vi "Write to Syslog.vi"(8 "error in (no error)":errorcluster, 10 "message":string, 11 "CIF Message Type":T1) -> (0 "error out":errorcluster)   [LabVIEW 2021, in "CIFLogs.lvlib"]
uses:
  CIFLogs.lvlib
  Typedef/Message Type.ctl
  <vilib>/CIF Foundation/CIF Utilities/Time/System Time/LabVIEW Time to TAI Time.vi
  Typedef/syslog facility.ctl
  Typedef/syslog priority.ctl
  <vilib>/CIF Foundation/CIF Utilities/Time/Time_CIF_U.lvlib
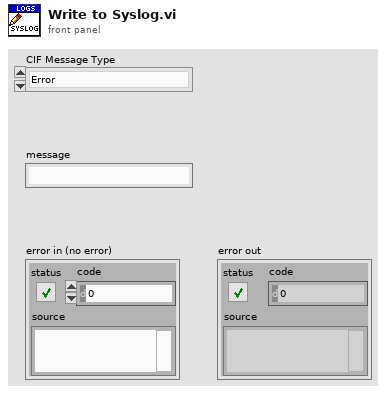
[diagram p1: front panel]
types:
  T1 = typedef "CIFLogs.lvlib/Message Type.ctl" = enum16{"Error", "Information", "Print Terminal", "Configuration"}
  T2 = typedef "CIFLogs.lvlib/syslog priority.ctl" = enum8{"emerg", "alert", "crit", "err", "warning", "notice", "info", "debug"}
  T3 = typedef "CIFLogs.lvlib/syslog facility.ctl" = enum16{"kern", "user", "mail", "daemon", "auth", "syslog", "lpr", "news", "uucp", "cron", "authpriv", "ftp", "rsrv1", "rsrv2", "rsrv3", "rsrv4", "local0", "local1", "local2", "local3", "local4", "local5", "local6", "local7"}
  T4 = enum16{"open", "replace", "create", "open or create", "replace or create", "replace or create with confirmation"}
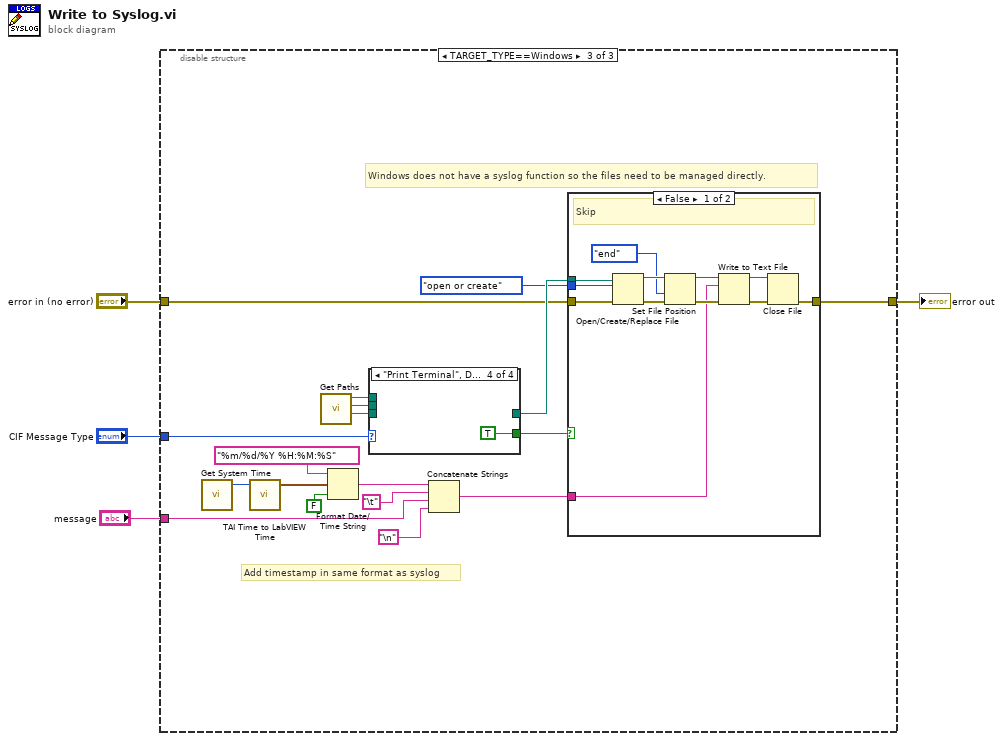
[diagram p0: block diagram]
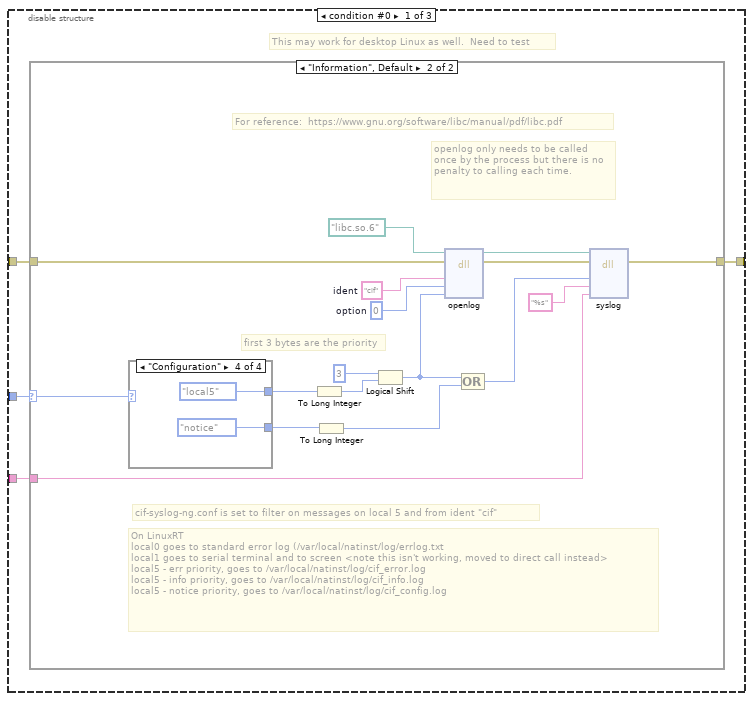
[diagram p2: hidden frame]
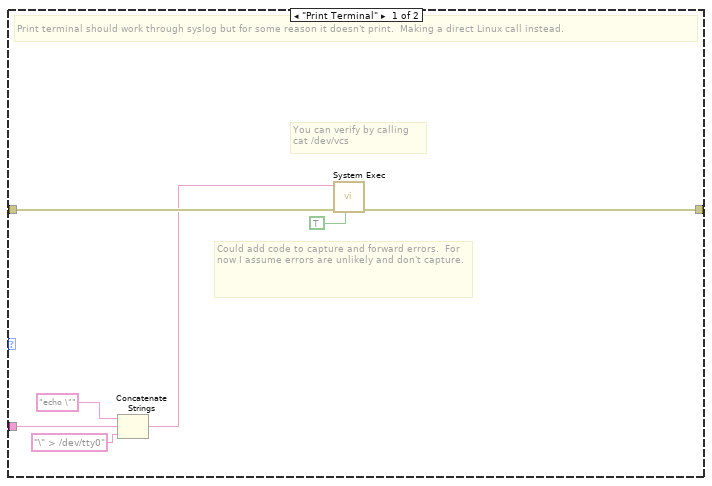
[diagram p3: hidden frame]
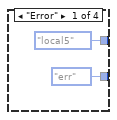
[diagram p4: hidden frame]
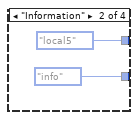
[diagram p5: hidden frame]
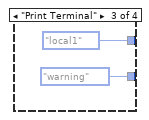
[diagram p6: hidden frame]
diagram:
  n1 = disable-structure shown="TARGET_TYPE==Windows" {
    disable-tunnel: "error in (no error)" -> [w8 w41 w46]
    disable-tunnel: [w7 w41 w47] -> w3
    disable-tunnel: "message" -> [w6 _ w54]
    disable-tunnel: "CIF Message Type" -> [w5 _ w52]
    frame condition #0 {
      # "This may work for desktop Linux as well.  Need to test"
      n2 = case shown="\"Information\", Default" w5 {
        selector: w5 -> [_ w16]
        tunnel: w8 -> [w15 w30]
        tunnel: [w14 w27] -> w7
        tunnel: w6 -> [w11 w17]
        frame "Print Terminal" {
          # "You can verify by calling \ncat /dev/vcs"
          # "Could add code to capture and forward errors.  For now I assume errors are unlikely and don't capture."
          # "Print terminal should work through syslog but for some reason it doesn't print.  Making a direct Linux call instead."
          n3 = Concatenate Strings("echo \"", w11, "\" > /dev/tty0") -> (w9:string)
          n4 = call <vilib>:"System Exec.vi"("run minimized? (F)"=TRUE, "error in (no error)"=w15, "command line"=w9) -> ("error out"=w14:errorcluster)  [unwired: 5 in, 3 out]
        }
        frame "Information", Default {
          w25 = 0  # option
          w26 = "cif"  # ident
          # "On LinuxRT\nlocal0 goes to standard error log (/var/local/natinst/log/errlog.txt\nlocal1 goes to serial terminal and to screen <note this isn't working, moved to direct call instead>\nlocal5 - err priority, goes to /var/local/natinst/log/cif_error.log\nlocal5 - info priority, goes to /var/local/natinst/log/cif_info.log\nlocal5 - notice priority, goes to /var/local/natinst/log/cif_config.log"
          # "first 3 bytes are the priority"
          # "cif-syslog-ng.conf is set to filter on messages on local 5 and from ident \"cif\""
          # "For reference:  https://www.gnu.org/software/libc/manual/pdf/libc.pdf"
          # "openlog only needs to be called once by the process but there is no penalty to calling each time."
          n5 = case shown="\"Configuration\"" w16 {
            tunnel: [syslog_facility."local5" ("Facility") syslog_facility."local5" ("Facility") syslog_facility."local1" ("Facility") syslog_facility."local5" ("Facility")] -> w24
            tunnel: [syslog_priority."err" ("Priority") syslog_priority."info" ("Priority") syslog_priority."warning" ("Priority") syslog_priority."notice" ("Priority")] -> w20
            frame "Error" {
            }
            frame "Information" {
            }
            frame "Print Terminal" {
            }
            frame "Configuration" {
            }
          }
          n6 = To Long Integer(number=w24) -> (32bit integer=w22:i32)
          n7 = To Long Integer(number=w20) -> (32bit integer=w19:i32)
          n8 = Logical Shift(y=i16 3 ("n"), x=w22) -> (x << y=w21:i32)
          n9 = dll-call lib="libc.so.6" fn="openlog"(path in=path "libc.so.6", error in=w30, "ident"=w26, "option"=w25, "facility"=w21) -> (path out=w29:path, error out=w28:errorcluster)  [unwired: 5 in]
          n10 = Compound Arithmetic op=OR(w21, w19) -> (w18:i32)
          n11 = dll-call lib="libc.so.6" fn="syslog"(path in=w29, error in=w28, "priority"=w18, "format"="%s", "message"=w17) -> (error out=w27:errorcluster)  [unwired: 5 in, 1 out]
        }
      }
    }
    frame condition #1 {
    }
    frame condition #2 (active) {
      # "Add timestamp in same format as syslog"
      # "Windows does not have a syslog function so the files need to be managed directly."
      n12 = call <vilib>:"Get System Time.vi"() -> ("Time (ns)"=w56:i64)  [unwired: 5 in]
      n13 = call <vilib>:"TAI Time to LabVIEW Time.vi"("TAI Time (ns)"=w56) -> ("LabVIEW Time (s)"=w57:timestamp)  [unwired: 4 in]
      n14 = call "Get Paths.vi"() -> ("Info Log"=w49:path, "Config Log"=w50:path, "Error Log"=w51:path)  [unwired: 9 in]
      n15 = Format Date/Time String(time format string (%c)="%m/%d/%Y %H:%M:%S", seconds (now)=w57, UTC format=FALSE) -> (date/time string=w55:string)
      n16 = case shown="\"Print Terminal\", Default" w52 {
        tunnel: w51 -> [_ _ w75 _]
        tunnel: w50 -> [_ w74 _ _]
        tunnel: w49 -> [w73 _ _ _]
        tunnel: [w73 w74 w75 _] -> w48
        tunnel: [_ _ _ TRUE] -> w43
        frame "Information" {
        }
        frame "Configuration" {
        }
        frame "Error" {
        }
        frame "Print Terminal", Default {
        }
      }
      n17 = Concatenate Strings(w55, "\t", w54, "\n") -> (w45:string)
      n18 = case shown="False" w43 {
        tunnel: w48 -> [w71 _]
        tunnel: [w63 w72] -> w47
        tunnel: w46 -> [w62 w72]
        tunnel: w45 -> [w61 _]
        tunnel: T4."open or create" ("operation (0:open)") -> [w60 _]
        frame False {
          # "Skip"
          n19 = Open/Create/Replace File(file path (use dialog)=w71, error in=w62, operation (0:open)=w60) -> (refnum out=w70:refnum<file>, error out=w69:errorcluster)  [unwired: 3 in, 1 out]
          n20 = Set File Position(refnum=w70, from (0:start)=enum16{"start", "end", "current"}."end", error in=w69) -> (refnum out=w67:refnum<file>, error out=w66:errorcluster)  [unwired: 1 in]
          n21 = Write to Text File(file (use dialog)=w67, text=w61, error in=w66) -> (refnum out=w65:refnum<file>, error out=w64:errorcluster)  [unwired: 1 in, 1 out]
          n22 = Close File(refnum=w65, error in=w64) -> (error out=w63:errorcluster)  [unwired: 1 out]
        }
        frame True {
        }
      }
    }
  }
  "error out" <- w3
